vi "Dump.vi"(8 "error in (no error)":errorcluster, 11 "skvc":string[][](array[string])) -> (0 "error out":errorcluster, 3 "Text":string)   [LabVIEW 2021, in "Config.lvlib"]
uses:
  Config.lvlib
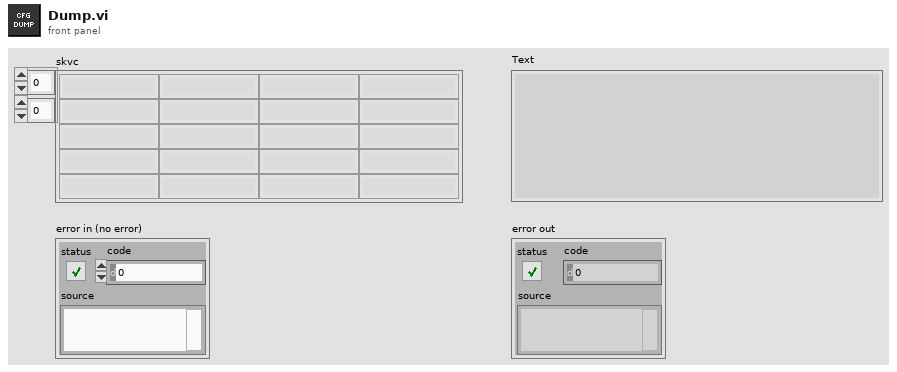
[diagram p1: front panel]
types:
  T1 = cluster{"Section":string, "Comment":string, "Keys":string[][]}[]
  T2 = cluster{"Section":string, "Comment":string, "Keys":string[][]}
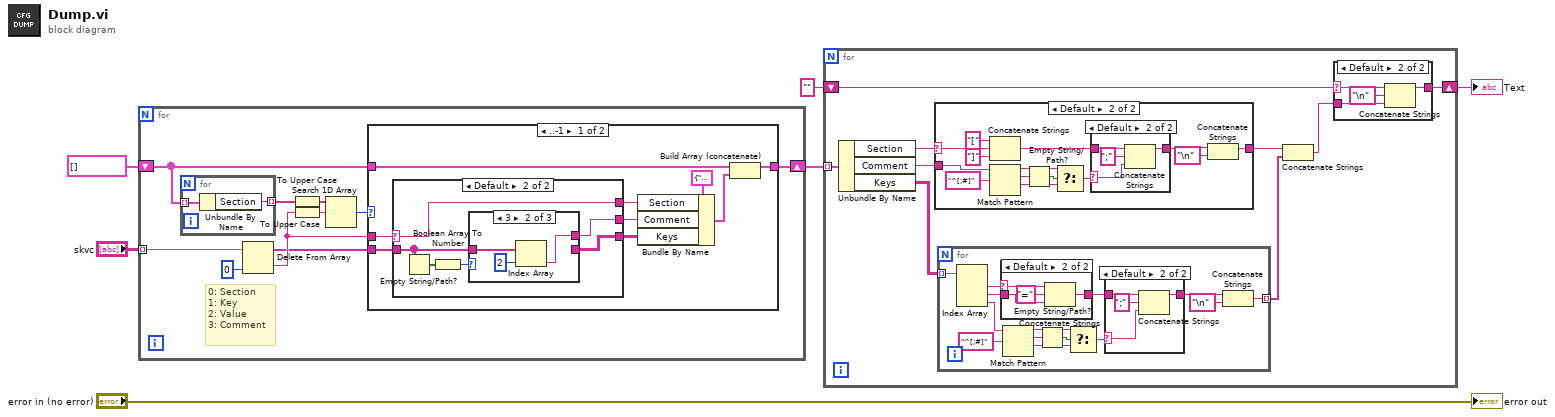
[diagram p0: block diagram]
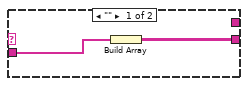
[diagram p2: hidden frame]
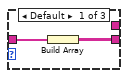
[diagram p3: hidden frame]
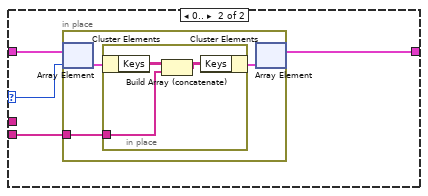
[diagram p5: hidden frame]
diagram:
  n1 = for {
    tunnel: "skvc" -> [w16] mode=indexing
    shift-right: [w7] -> w1
    shift-left: T1 [] ("Sections") -> [w10]
    # "0: Section\n1: Key\n2: Value\n3: Comment"
    n2 = for {
      tunnel: w10 -> [w50] mode=indexing
      tunnel: [w49] -> w14 mode=indexing
      n3 = Unbundle By Name(w50) -> ("Section"=w49:string)
    }
    n4 = Delete From Array(array=w16, index=0) -> (deleted portion=w9:string, array with subset deleted=w8:string[])  [unwired: 1 in]
    n5 = To Upper Case(1:w14) -> (0:w12:string[])
    n6 = To Upper Case(1:w9) -> (0:w13:string)
    n7 = Search 1D Array(1D array=w12, element=w13) -> (index of element=w11:i32)  [unwired: 1 in]
    n8 = case shown="..-1" w11 {
      selector: w11 -> [_ w41]
      tunnel: w10 -> [w25 w42]
      tunnel: [w23 w39] -> w7
      tunnel: w9 -> [w17 _]
      tunnel: w8 -> [w21 w40]
      frame ..-1 {
        n9 = case shown="Default" w17 {
          selector: w17 -> [_ w28]
          tunnel: w21 -> [w27 w31]
          tunnel: [w26 w30] -> w20
          tunnel: [_ w29] -> w19
          tunnel: [_ w28] -> w18
          frame "" {
            n10 = Build Array(w27) -> (w26:string[][])
          }
          frame Default {
            n11 = Empty String/Path?(string/path=w31) -> (empty?=w33:bool[])
            n12 = Boolean Array To Number(Boolean array=w33) -> (number=w32:u32)
            n13 = case shown="3" w32 {
              tunnel: w31 -> [w35 w38 _]
              tunnel: [w34 _ _] -> w30
              tunnel: [_ w37 _] -> w29
              frame Default {
                n14 = Build Array(w35) -> (w34:string[][])
              }
              frame 3 {
                n15 = Index Array(array=w38, index=2) -> (element=w37:string)
              }
              frame 7 {
                # "All empty"
              }
            }
          }
        }
        n16 = Bundle By Name(cluster=T2 {"Section"="", "Comment"="", "Keys"=[]}, "Section"=w18, "Comment"=w19, "Keys"=w20) -> (w22:T2)
        n17 = Build Array (concatenate)(w25, w22) -> (w23:T1)
      }
      frame 0.. {
        n18 = in-place {
          in-place-border: w40 -> [w44]
          n19 = in-place-array #1(w42, w41) -> (w45:T2)
          n20 = in-place {
            in-place-border: w44 -> [w46]
            n21 = in-place-cluster #2(w45) -> ("Keys"=w48:string[][])
            n22 = Build Array (concatenate)(w48, w46) -> (w47:string[][])
            n23 = in-place-cluster #2("Keys"=w47) -> (w43:T2)
          }
          n24 = in-place-array #1(w43) -> (w39:T1)  [unwired: 1 out]
        }
      }
    }
  }
  n25 = for {
    tunnel: w1 -> [w59] mode=indexing
    shift-right: [w52] -> w6
    shift-left: "" -> [w51]
    n26 = Unbundle By Name(w59) -> ("Section"=w58:string, "Comment"=w57:string, "Keys"=w56:string[][])
    n27 = case shown="Default" w58 {
      selector: w58 -> [_ w101]
      tunnel: w57 -> [_ w91]
      tunnel: [_ w88] -> w54
      frame "" {
      }
      frame Default {
        n28 = Concatenate Strings("[" ("string"), w101, "]" ("string")) -> (w92:string)
        n29 = Match Pattern(string=w91, regular expression="^[;#]") -> (before substring=w97:string, match substring=w95:string, after substring=w96:string)  [unwired: 1 in, 1 out]
        n30 = Empty String/Path?(string/path=w95) -> (empty?=w94:bool)
        n31 = Select(t=w97, s=w94, f=w96) -> (s? t:f=w93:string)
        n32 = case shown="Default" w93 {
          selector: w93 -> [_ w105]
          tunnel: w92 -> [w102 w104]
          tunnel: [w102 w103] -> w89
          frame "" {
          }
          frame Default {
            n33 = Concatenate Strings(w104, ";" ("string"), w105) -> (w103:string)
          }
        }
        n34 = Concatenate Strings(w89, "\n" ("string")) -> (w88:string)
      }
    }
    n35 = for {
      tunnel: w56 -> [w78] mode=indexing
      tunnel: [w65] -> w55 mode=indexing
      n36 = Index Array(array=w78) -> (element #1=w71:string, element #2=w70:string, element #3=w68:string)  [unwired: 3 in]
      n37 = case shown="Default" w71 {
        selector: w71 -> [_ w82]
        tunnel: w70 -> [_ w80]
        tunnel: [_ w79] -> w69
        frame "" {
        }
        frame Default {
          n38 = Concatenate Strings(w82, "=" ("string"), w80) -> (w79:string)
        }
      }
      n39 = Match Pattern(string=w68, regular expression="^[;#]") -> (before substring=w73:string, match substring=w75:string, after substring=w74:string)  [unwired: 1 in, 1 out]
      n40 = Empty String/Path?(string/path=w75) -> (empty?=w76:bool)
      n41 = Select(t=w73, s=w76, f=w74) -> (s? t:f=w77:string)
      n42 = case shown="Default" w77 {
        selector: w77 -> [_ w86]
        tunnel: w69 -> [w83 w85]
        tunnel: [w83 w84] -> w67
        frame "" {
        }
        frame Default {
          n43 = Concatenate Strings(w85, ";" ("string"), w86) -> (w84:string)
        }
      }
      n44 = Concatenate Strings(w67, "\n" ("string")) -> (w65:string)
    }
    n45 = Concatenate Strings(w54, w55) -> (w53:string)
    n46 = case shown="Default" w51 {
      selector: w51 -> [_ w63]
      tunnel: [w60 w64] -> w52
      tunnel: w53 -> [w60 w61]
      frame "" {
      }
      frame Default {
        n47 = Concatenate Strings(w63, "\n" ("string"), w61) -> (w64:string)
      }
    }
  }
  "Text" <- w6
  "error out" <- "error in (no error)"
